vi "TagMetadataToImage.vi"(8 "error in (no error)":errorcluster, 10 "Image In":T1, 11 "StageController in":refnum<class "StageController.lvclass">) -> (0 "error out":errorcluster, 2 "Image Out":T1, 3 "StageController out":refnum<class "StageController.lvclass">)   [LabVIEW 2020, in "StageController.lvlib" / "StageController.lvclass"]
uses:
  StageController.lvclass
  <vilib>/vision/Image Controls.llb/IMAQ Image.ctl
  StageController.lvclass/StageController.ctl
  Model/Hardware Abstraction Layer/Component/GenericActor/GenericActor/GenericController.lvclass
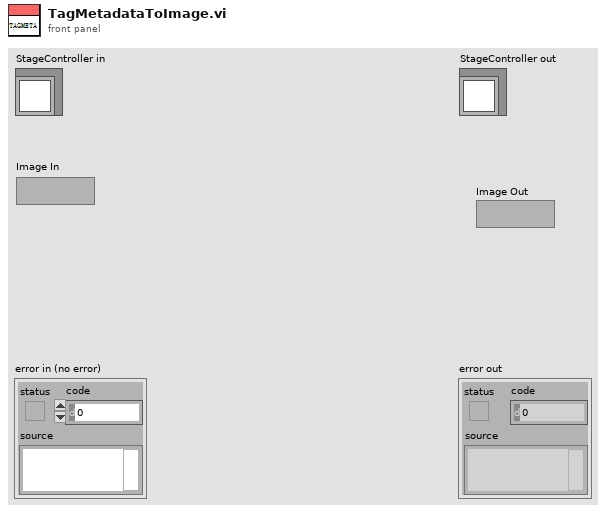
[diagram p1: front panel]
types:
  T1 = typedef "IMAQ Image.ctl" = refnum<image>
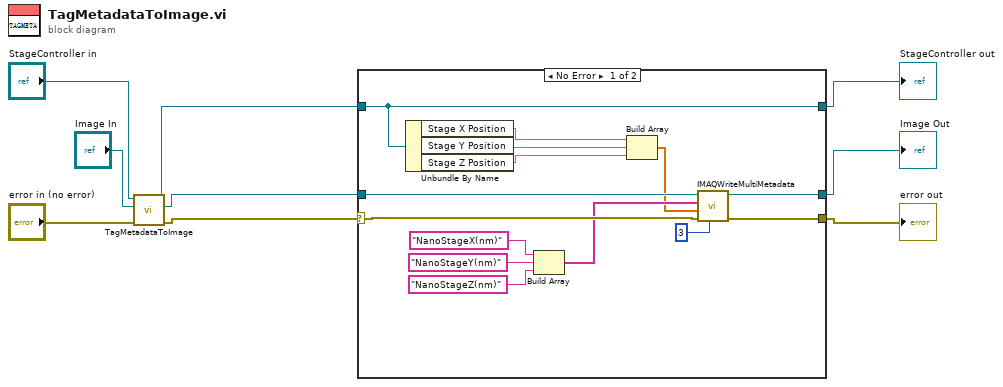
[diagram p0: block diagram]
diagram:
  n1 = call-parent "TagMetadataToImage.vi"("error in (no error)"="error in (no error)", "Image In"="Image In", "GenericController in"="StageController in") -> ("error out"=w6:errorcluster, "Image Out"=w5:T1, "GenericController out"=w4:refnum<class "StageController.lvclass">)  [unwired: 6 in]
  n2 = case shown="No Error" w6 {
    selector: w6 -> [w23 w26]
    tunnel: [w21 w26] -> w1
    tunnel: w5 -> [w22 w24]
    tunnel: [w10 w25] -> w3
    tunnel: w4 -> [w10 w25]
    tunnel: [w20 w24] -> w2
    frame No Error {
      n3 = Unbundle By Name(w10) -> ("Stage X Position"=w14:dbl, "Stage Y Position"=w13:dbl, "Stage Z Position"=w12:dbl)
      n4 = Build Array("NanoStageX(nm)" ("Key"), "NanoStageY(nm)" ("Key"), "NanoStageZ(nm)" ("Key")) -> (w15:string[])
      n5 = Build Array(w14, w13, w12) -> (w11:dbl[])
      n6 = call "IMAQWriteMultiMetadata.vi"("precision (6)"=i16 3, "error in (no error)"=w23, "Values"=w11, "Keys"=w15, "Image In"=w22) -> ("error out"=w21:errorcluster, "Image Out"=w20:T1)  [unwired: 5 in]
    }
    frame Error {
    }
  }
  "error out" <- w1
  "StageController out" <- w3
  "Image Out" <- w2
